vi "visionNut.vi"(8 "Error In":errorcluster, 11 "Aim_Color":string="Default") -> (0 "Error Out":errorcluster, 2 "Left | right":bool, 3 "Nut_position":string)   [LabVIEW 2019]
uses:
  WSCbot_V3_Toolkit.lvlibp
panel:
  out "Classes (Color Classification 1)":string[](array[string])
  out "position_index":i32
  in  "Stop Button":bool
  out "Image Out":T1(plugin-control)
  out "original":T1(plugin-control)
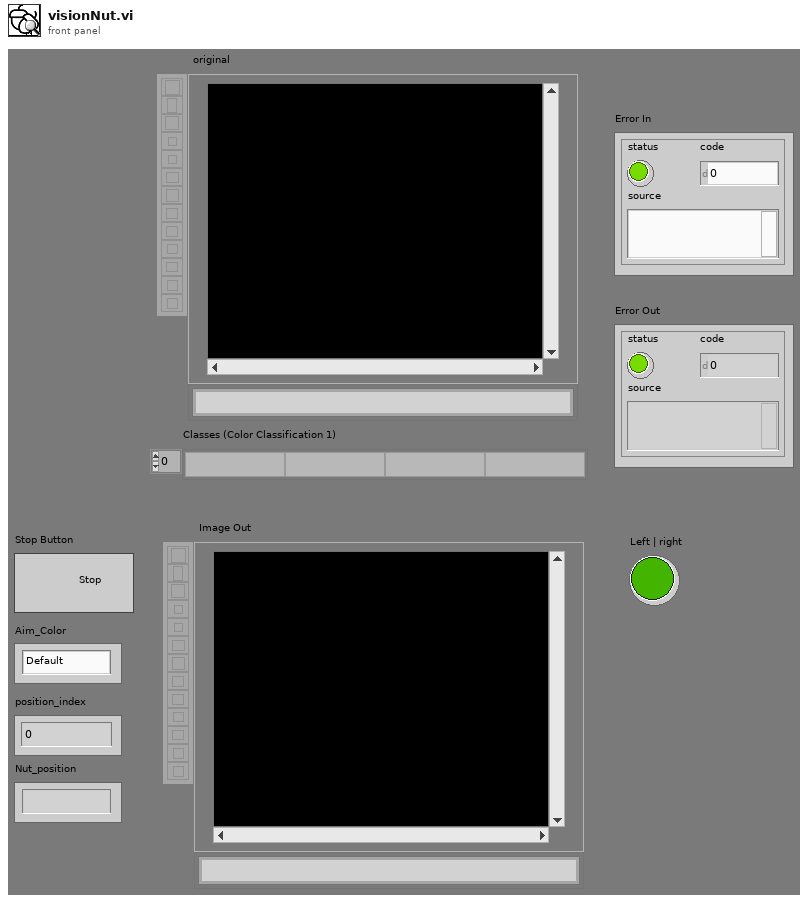
[diagram p1: front panel]
types:
  T1 = typedef "IMAQ Image.ctl" = refnum<image>
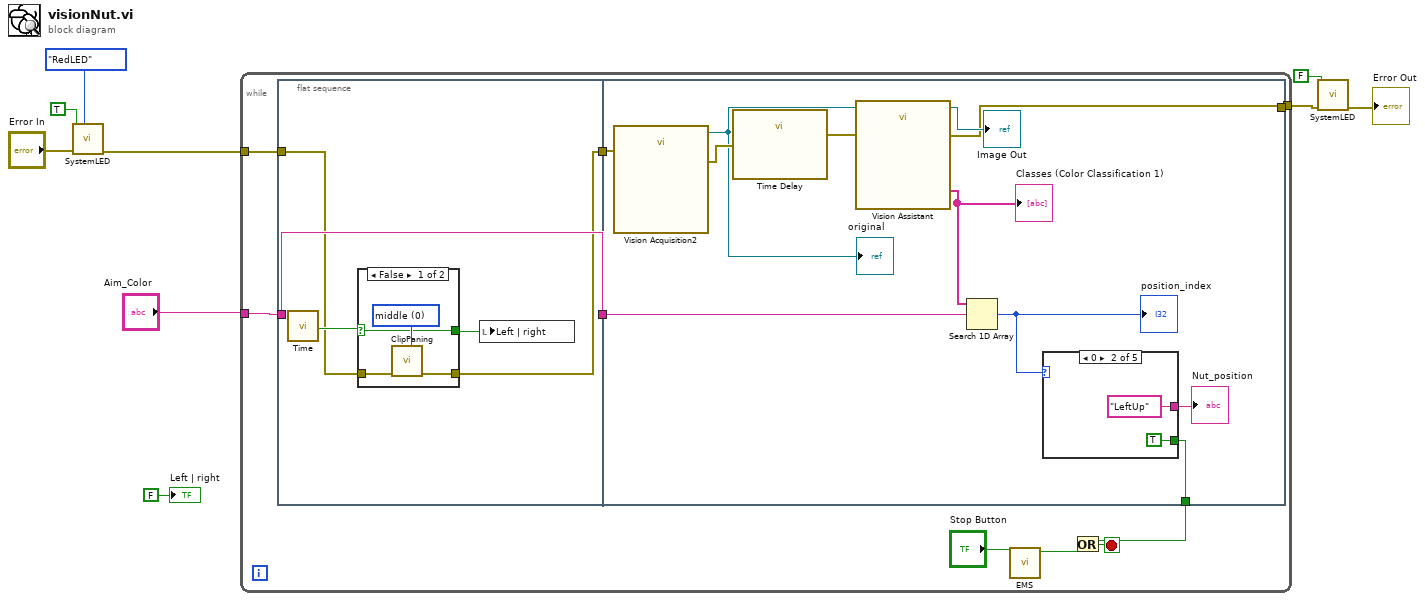
[diagram p0: block diagram]
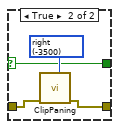
[diagram p2: hidden frame]
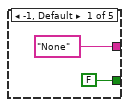
[diagram p3: hidden frame]
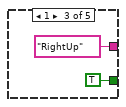
[diagram p4: hidden frame]
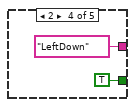
[diagram p5: hidden frame]
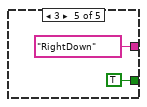
[diagram p6: hidden frame]
diagram:
  n1 = call "SystemLED.vi"("SelectColor"=enum16{"RedLED", "GreenLED", "YellowLED"}."RedLED", "error in"="Error In", "Set"=TRUE) -> ("error out"=w2:errorcluster)  [unwired: 8 in]
  n2 = while {
    tunnel: "Aim_Color" -> [w18]
    tunnel: w2 -> [w13]
    tunnel: [w12] -> w1
    stop <- w16 stop-if-true
    n3 = flat-sequence {
      tunnel: w13 -> [w20]
      tunnel: w18 -> [w23]
      tunnel: [w23] -> w11
      tunnel: [w19] -> w10
      tunnel: [w36] -> w14
      tunnel: [w35] -> w12
      tunnel: w11 -> [w40]
      tunnel: w10 -> [w34]
      frame #0 {
        n4 = call "Time"() -> ("Time has Elapsed"=w21:bool)  [unwired: 12 in, 7 out]
        n5 = case shown="False" w21 {
          selector: w21 -> [w26 w30]
          tunnel: [w26 w30] -> w22
          tunnel: w20 -> [w25 w29]
          tunnel: [w24 w28] -> w19
          frame False {
            w27 = 0 items=["left"=2100, "right"=-3500, "lock screw"=1345, "lock_nut"=1167, "middle"=0] ("location")
            n6 = call "ClipPaning.vi"("Error In"=w25, "location"=w27) -> ("Error Out"=w24:errorcluster)  [unwired: 8 in]
          }
          frame True {
            w31 = -3500 items=["left"=2100, "right"=-3500, "lock screw"=1345, "lock_nut"=1167, "middle"=0] ("location")
            n7 = call "ClipPaning.vi"("Error In"=w29, "location"=w31) -> ("Error Out"=w28:errorcluster)  [unwired: 8 in]
          }
        }
        n8 = local write "Left | right"(w22) -> ()
      }
      frame #1 {
        n9 = call "Vision Acquisition2"("error in"=w34) -> ("Image Out"=w32:T1, "error out"=w33:errorcluster)  [unwired: 25 in]
        "original" <- w32
        n10 = call "Time Delay"("error in (no error)"=w33) -> ("error out"=w39:errorcluster)  [unwired: 10 in]
        n11 = call "Vision Assistant"("Image In"=w32, "error in"=w39) -> ("Image Out"=→"Image Out":T1, "Classes (Color Classification 1)"=w41:string[], "error out"=w35:errorcluster)  [unwired: 23 in]
        "Classes (Color Classification 1)" <- w41
        n12 = Search 1D Array(1D array=w41, element=w40) -> (index of element=w38:i32)  [unwired: 1 in]
        "position_index" <- w38
        n13 = case shown="0" w38 {
          tunnel: ["None" "LeftUp" "RightUp" "LeftDown" "RightDown"] -> w37
          tunnel: [FALSE TRUE TRUE TRUE TRUE] -> w36
          frame -1, Default {
          }
          frame 0 {
          }
          frame 1 {
          }
          frame 2 {
          }
          frame 3 {
          }
        }
        "Nut_position" <- w37
      }
    }
    n14 = call "EMS.vi"("ProgramStop"="Stop Button") -> ("EMS"=w15:bool)  [unwired: 9 in, 1 out]
    n15 = Or(x=w14, y=w15) -> (x .or. y?=w16:bool)
  }
  n16 = call "SystemLED.vi"("error in"=w1, "Set"=FALSE) -> ("error out"=→"Error Out":errorcluster)  [unwired: 9 in]
  "Left | right" <- FALSE ("Left | right")
